vi "SystemController.GetConfiguration.vi"(8 "error in (no error)":errorcluster, 11 "SystemController":refnum<class "SystemController.lvclass">) -> (0 "error out":errorcluster, 2 "Configuration":T1={"Camera"={"Simulate Camera"=FALSE, "IMAQ Camera"={"Camera Interface Name"="", "Number of Buffers"=0, "Image Name"="", "Image Type"=0}, "Simulated Camera Image"=path ""}, "Find Eyes"=FALSE, "Acquisition Rate (ms)"=500} {"Camera"."IMAQ Camera"."Image Type" items=["Grayscale (U8)", "Grayscale (I16)", "Grayscale (SGL)", "Complex (CSG)", "RGB (U32)", "HSL (U32)", "RGB (U64)", "Grayscale (U16)"]}, 3 "SystemController out":refnum<class "SystemController.lvclass">)   [LabVIEW 2017, in "SystemController.lvclass"]
doc: "---------------------------------------------------------------\nJKI State Machine Objects™\nhttp://jki.net/state-machine-objects/\nCopyright (C) 2005-2015, JKI <info@jki.net>\nALL RIGHTS RESERVEDJKI State Machine Objects (SMO) 1.0.0.5\nJKI - JKI\nCopyright (c) 2016, JKI"
uses:
  SystemController.lvclass
  Typedefs/Configuration--Cluster.ctl
  Typedefs/CameraConfig--Cluster.ctl
  Camera/Camera_IMAQdx_class/typedefs/Configuration--Cluster.ctl
  SystemController.lvclass/SystemController.ctl
  Camera/Camera_IMAQdx_class/Camera_IMAQdx.lvclass
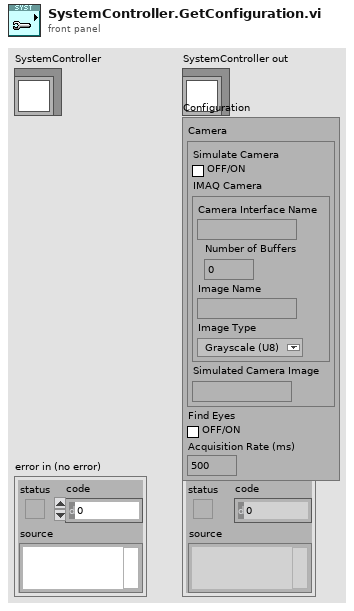
[diagram p1: front panel]
types:
  T1 = typedef "SystemController.lvclass/Configuration--Cluster.ctl" = cluster{"Camera":T2, "Find Eyes":bool, "Acquisition Rate (ms)":i32}
  T2 = typedef "SystemController.lvclass/CameraConfig--Cluster.ctl" = cluster{"Simulate Camera":bool, "IMAQ Camera":T3, "Simulated Camera Image":path}
  T3 = typedef "Camera_IMAQdx.lvclass/Configuration--Cluster.ctl" = cluster{"Camera Interface Name":string, "Number of Buffers":u32, "Image Name":string, "Image Type":T4}
  T4 = typedef "Image Type" = u32
  T5 = typedef "SystemController.lvclass/PrivateData--Ref.ctl" = refnum<data-value>
  T6 = typedef "SystemController.lvclass/PrivateData--Cluster.ctl" = cluster{"Configuration":T1, "Dependencies":T7, "ProcessedImage":T8, "Public Events":T9}
  T7 = typedef "SystemController.lvclass/Dependencies--Cluster.ctl" = cluster{"Camera":refnum<class "Camera.lvclass">, "ImageFacialDetection":refnum<class "ImageFacialDetection.lvclass">}
  T8 = typedef "IMAQ Image.ctl" = refnum<image>
  T9 = typedef "SystemController.lvclass/PublicEvents--Cluster.ctl" = cluster{"UIClosed":refnum<user-event>}
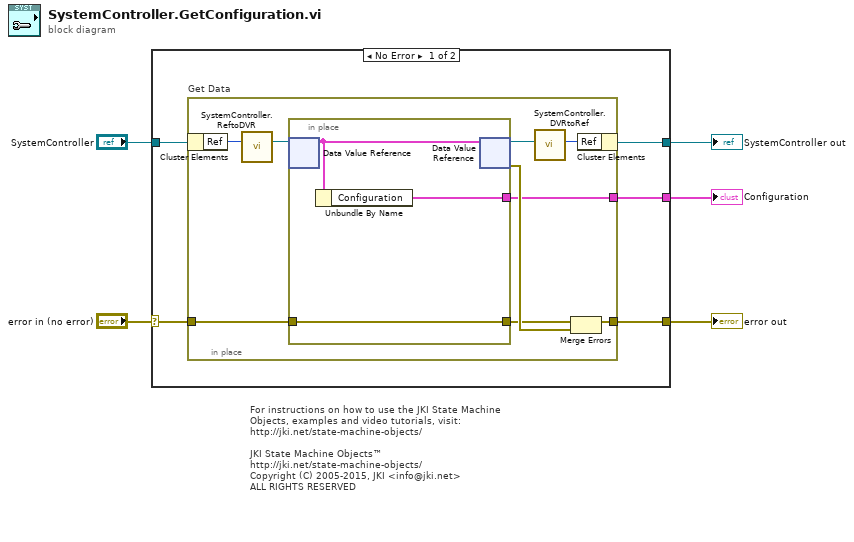
[diagram p0: block diagram]
diagram:
  # "For instructions on how to use the JKI State Machine Objects, examples and video tutorials, visit:\nhttp://jki.net/state-machine-objects/\n\nJKI State Machine Objects™\nhttp://jki.net/state-machine-objects/\nCopyright (C) 2005-2015, JKI <info@jki.net>\nALL RIGHTS RESERVED"
  n1 = case shown="No Error" "error in (no error)" {
    selector: "error in (no error)" -> [w9 w23]
    tunnel: "SystemController" -> [w10 w24]
    tunnel: [w7 w23] -> w4
    tunnel: [w8 w24] -> w3
    tunnel: [w6 _] -> w1
    frame No Error {
      n2 = in-place "Get Data" {
        in-place-border: w9 -> [w19]
        in-place-border: [w16] -> w7
        in-place-border: [w15] -> w6
        n3 = in-place-cluster #1(w10) -> ("Ref"=w14:u32)
        n4 = call "SystemController.ReftoDVR.vi"("Ref"=w14) -> ("Ref"=w13:T5)  [unwired: 10 in]
        n5 = in-place {
          in-place-border: w19 -> [w21]
          in-place-border: [w21] -> w17
          in-place-border: [w20] -> w15
          n6 = in-place-dvr #2(w13) -> (w22:T6)  [unwired: 1 out]
          n7 = Unbundle By Name(w22) -> ("Configuration"=w20:T1)
          n8 = in-place-dvr #2(w22) -> (w12:T5, w18:errorcluster)
        }
        n9 = call "SystemController.DVRtoRef.vi"("Ref"=w12) -> ("Ref"=w11:u32)  [unwired: 10 in]
        n10 = Merge Errors(w17, w18) -> (w16:errorcluster)
        n11 = in-place-cluster #1("Ref"=w11) -> (w8:refnum<class "SystemController.lvclass">)
      }
    }
    frame Error {
    }
  }
  "error out" <- w4
  "SystemController out" <- w3
  "Configuration" <- w1
